vi "Create Random Array.vi"(1 "Array Size":i32) -> (0 "Random Array Out":dbl[](array[numeric]))   [LabVIEW 2015]
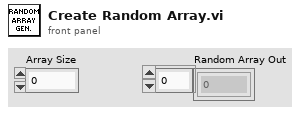
[diagram p1: front panel]
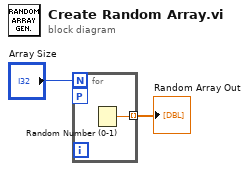
[diagram p0: block diagram]
diagram:
  n1 = for {
    N: "Array Size" -> [_]
    tunnel: [w3] -> w1 mode=indexing
    workers-P: _ -> [_]
    n2 = Random Number (0-1)() -> (number: 0 to 1=w3:dbl)
  }
  "Random Array Out" <- w1
